vi "RT Loop Stop.vi"() -> ()   [LabVIEW 2018]
panel:
  in  "RT Loop Stop":bool
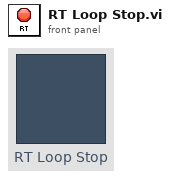
[diagram p1: front panel]
diagram:
